vi "Load VI.vi"(8 "error in (no error)":errorcluster, 11 "y":string) -> (0 "error out":errorcluster, 3 "VI out":refnum<vi>)   [LabVIEW 2025, in "Scripting Server.lvlib" / "Tools.lvlib"]
uses:
  Tools/Tools.lvlib
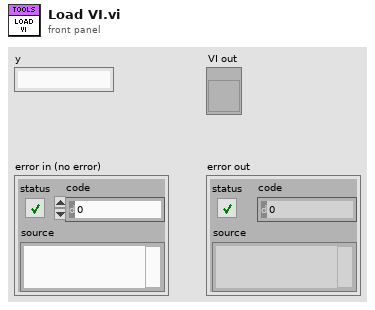
[diagram p1: front panel]
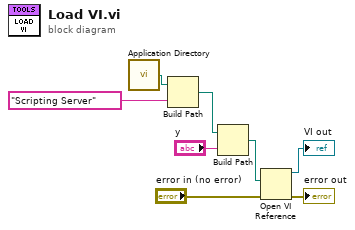
[diagram p0: block diagram]
diagram:
  n1 = call <vilib>:"Application Directory.vi"() -> ("Application Directory"=w5:path)
  n2 = Build Path(base path=w5, name or relative path="Scripting Server" ("format string")) -> (appended path=w6:path)
  n3 = Build Path(base path=w6, name or relative path="y") -> (appended path=w4:path)
  n4 = Open VI Reference(vi path=w4, error in (no error)="error in (no error)") -> (vi reference=→"VI out":refnum<vi>, error out=→"error out":errorcluster)  [unwired: 4 in]
